vi "set 站号.vi"(8 "error in (no error)":errorcluster caption="错误输入（无错误）", 10 "站号":u8, 11 "上位机 输入":refnum<class "上位机.lvclass">) -> (0 "error out":errorcluster caption="错误输出", 3 "上位机 输出":refnum<class "上位机.lvclass">)   [LabVIEW 2015, in "上位机.lvlib" / "上位机.lvclass"]
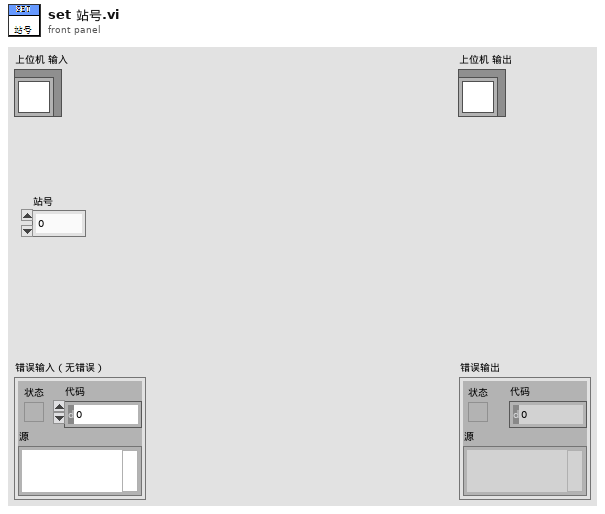
[diagram p1: front panel]
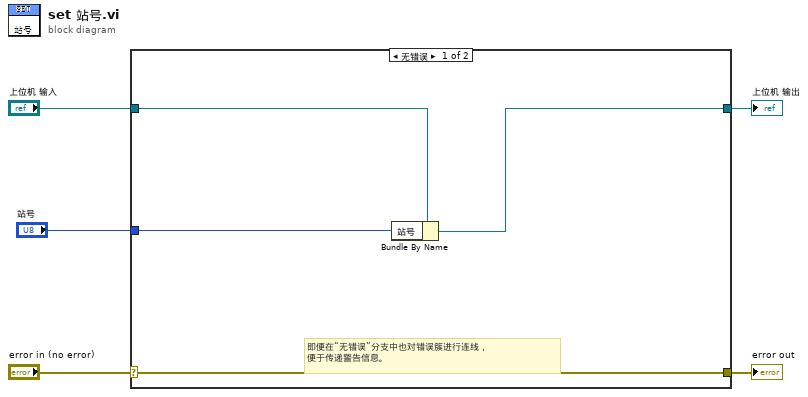
[diagram p0: block diagram]
diagram:
  n1 = case shown="无错误" "error in (no error)" {
    selector: "error in (no error)" -> [w9 w11]
    tunnel: [w9 w11] -> w4
    tunnel: [w7 w10] -> w2
    tunnel: "上位机 输入" -> [w8 w10]
    tunnel: "站号" -> [w6 _]
    frame No Error {
      # "即便在“无错误”分支中也对错误簇进行连线，\n便于传递警告信息。"
      n2 = Bundle By Name(cluster=w8, "站号"=w6) -> (w7:refnum<class "上位机.lvclass">)
    }
    frame Error {
    }
  }
  "error out" <- w4
  "上位机 输出" <- w2
